vi "buttonXMLExpression.vi"(8 "preValue":string, 9 "index":i32=5, 10 "xmlParser 0":string[](array[string]), 11 "String 4":string) -> (1 "stringFilter2":string, 2 "stringFilter1":string, 3 "buttonXMLExpression":string)   [LabVIEW 2018]
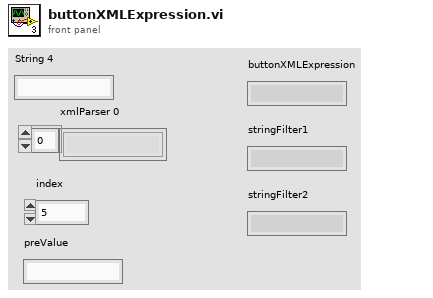
[diagram p1: front panel]
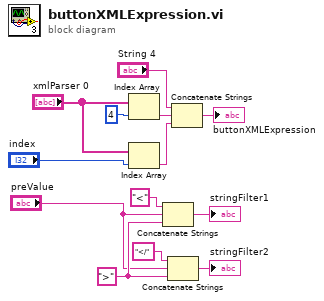
[diagram p0: block diagram]
diagram:
  w11 = ">" ("string")
  n1 = Index Array(array="xmlParser 0", index=4) -> (element=w3:string)
  n2 = Index Array(array="xmlParser 0", index="index") -> (element=w5:string)
  n3 = Concatenate Strings("<" ("string"), "preValue", w11) -> (→"stringFilter1":string)
  n4 = Concatenate Strings("</" ("string"), "preValue", w11) -> (→"stringFilter2":string)
  n5 = Concatenate Strings("String 4", w3, w5) -> (→"buttonXMLExpression":string)
